vi "createElement.vi"(6 "collectionInfo":T1, 8 "error in (no error)":errorcluster, 9 "elementBasicType":string, 10 "elementName":string, 11 "ElementFactory in":refnum<class "ElementFactory.lvclass">) -> (0 "error out":errorcluster, 2 "element":refnum<class "Element.lvclass">, 3 "ElementFactory out":refnum<class "ElementFactory.lvclass">)   [LabVIEW 2016, in "ElementFactory.lvclass"]
uses:
  ElementFactory.lvclass
  Element/Element.lvclass
  Typedefs/CollectionInfo.ctl
  Elements/Primitive/Primitive.lvclass
  D:/Code/ts_SALLabVIEW/SALTypeGenerator/Element/Element.lvclass
  Elements/Short/Short.lvclass
  D:/Code/ts_SALLabVIEW/SALTypeGenerator/Elements/Primitive/Primitive.lvclass
  Elements/Long/Long.lvclass
  Elements/LongLong/LongLong.lvclass
  Elements/UnsignedShort/UnsignedShort.lvclass
  Elements/UnsignedLong/UnsignedLong.lvclass
  Elements/UnsignedLongLong/UnsignedLongLong.lvclass
  Elements/Float/Float.lvclass
  Elements/Double/Double.lvclass
  Elements/Char/Char.lvclass
  Elements/Boolean/Boolean.lvclass
  Elements/String/String.lvclass
  Elements/String/String.lvclass/String.ctl
  Elements/Array/Array.lvclass
  Elements/Array/Array.lvclass/Array.ctl
  Element/Element.lvclass/Element.ctl
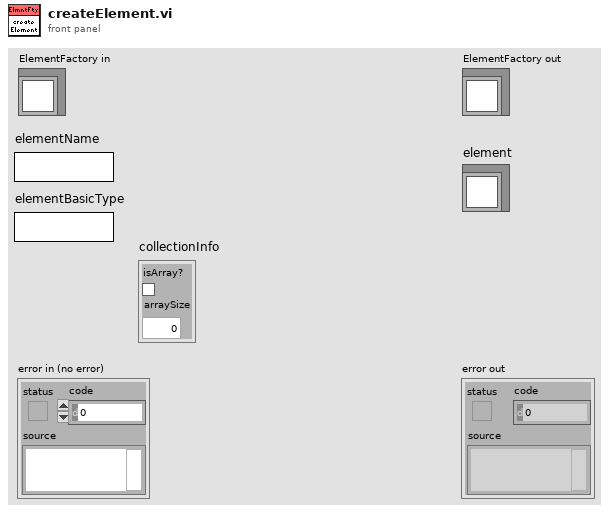
[diagram p1: front panel]
types:
  T1 = typedef "CollectionInfo.ctl" = cluster{"isArray?":bool, "arraySize":u16}
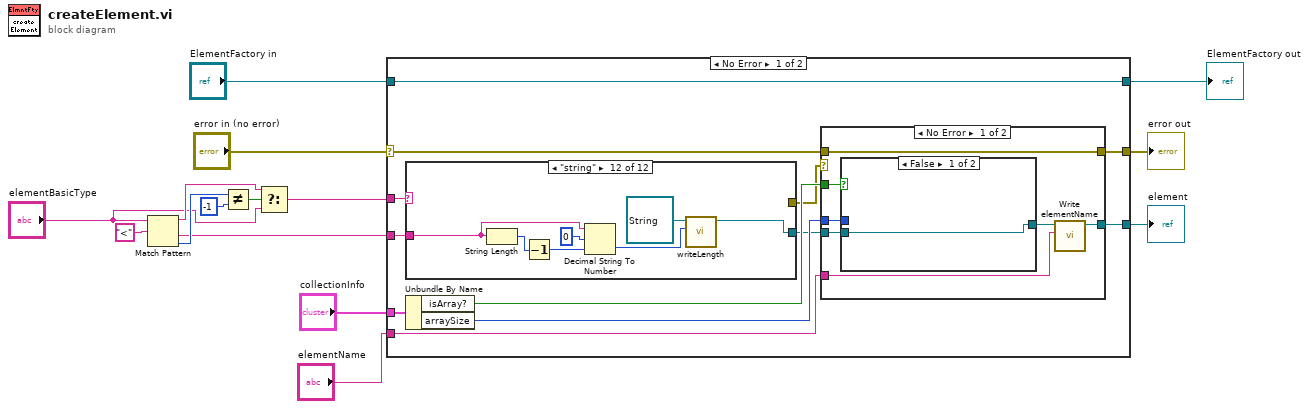
[diagram p0: block diagram]
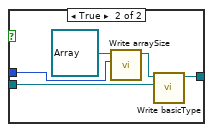
[diagram p2: hidden frame]
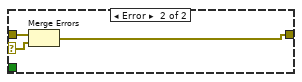
[diagram p3: hidden frame]
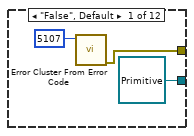
[diagram p4: hidden frame]
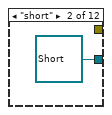
[diagram p5: hidden frame]
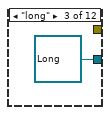
[diagram p6: hidden frame]
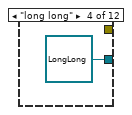
[diagram p7: hidden frame]
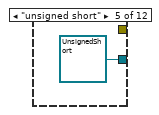
[diagram p8: hidden frame]
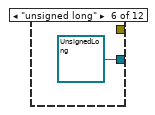
[diagram p9: hidden frame]
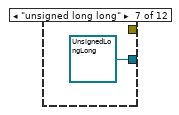
[diagram p10: hidden frame]
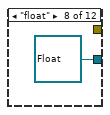
[diagram p11: hidden frame]
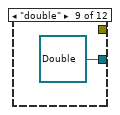
[diagram p12: hidden frame]
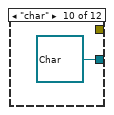
[diagram p13: hidden frame]
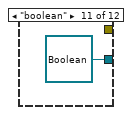
[diagram p14: hidden frame]
diagram:
  n1 = Match Pattern(string="elementBasicType", regular expression="<") -> (before substring=w4:string, after substring=w1:string, offset past match=w7:i32)  [unwired: 1 in, 1 out]
  n2 = Not Equal?(x=w7, y=-1) -> (x != y?=w5:bool)
  n3 = Select(t=w4, s=w5, f="elementBasicType") -> (s? t:f=w2:string)
  n4 = case shown="No Error" "error in (no error)" {
    selector: "error in (no error)" -> [w20 w65]
    tunnel: [w19 w65] -> w9
    tunnel: [w27 w64] -> w14
    tunnel: "ElementFactory in" -> [w27 w64]
    tunnel: w2 -> [w25 _]
    tunnel: "collectionInfo" -> [w26 _]
    tunnel: [w18 _] -> w13
    tunnel: "elementName" -> [w17 _]
    tunnel: w1 -> [w16 _]
    frame No Error {
      n5 = case shown="\"string\"" w25 {
        tunnel: [refnum<class "Primitive.lvclass"> refnum ("Boolean.lvclass") refnum<class "Short.lvclass"> refnum ("Short.lvclass") refnum<class "Long.lvclass"> refnum ("Long.lvclass") refnum<class "LongLong.lvclass"> refnum ("LongLong.lvclass") refnum<class "UnsignedShort.lvclass"> refnum ("UnsignedShort.lvclass") refnum<class "UnsignedLong.lvclass"> refnum ("UnsignedLong.lvclass") refnum<class "UnsignedLongLong.lvclass"> refnum ("UnsignedLongLong.lvclass") refnum<class "Float.lvclass"> refnum ("Float.lvclass") refnum<class "Double.lvclass"> refnum ("Double.lvclass") refnum<class "Char.lvclass"> refnum ("Char.lvclass") refnum<class "Boolean.lvclass"> refnum ("Boolean.lvclass") w58] -> w22
        tunnel: [w45 _ _ _ _ _ _ _ _ _ _ _] -> w21
        tunnel: w16 -> [_ _ _ _ _ _ _ _ _ _ _ w61]
        frame "False", Default {
          n6 = call <vilib>:"Error Cluster From Error Code.vi"("error code (0)"=5107) -> ("error out"=w45:errorcluster)  [unwired: 8 in]
        }
        frame "short" {
        }
        frame "long" {
        }
        frame "long long" {
        }
        frame "unsigned short" {
        }
        frame "unsigned long" {
        }
        frame "unsigned long long" {
        }
        frame "float" {
        }
        frame "double" {
        }
        frame "char" {
        }
        frame "boolean" {
        }
        frame "string" {
          n7 = String Length(string=w61) -> (length=w63:i32)
          n8 = Decrement(x=w63) -> (x-1=w62:i32)
          n9 = Decimal String To Number(string=w61, offset=0, default (0L)=w62) -> (number=w57:i32)  [unwired: 1 out]
          n10 = call "writeLength.vi"("Length"=w57, "String in"=refnum<class "String.lvclass"> refnum ("String.lvclass")) -> ("String out"=w58:refnum<class "String.lvclass">)  [unwired: 9 in]
        }
      }
      n11 = Unbundle By Name(w26) -> ("isArray?"=w23:bool, "arraySize"=w24:u16)
      n12 = case shown="No Error" w21 {
        selector: w21 -> [_ w42]
        tunnel: w24 -> [w34 _]
        tunnel: w23 -> [w33 _]
        tunnel: w22 -> [w32 _]
        tunnel: w20 -> [w31 w43]
        tunnel: [w31 w41] -> w19
        tunnel: [w29 _] -> w18
        tunnel: w17 -> [w28 _]
        frame No Error {
          n13 = case shown="False" w33 {
            tunnel: w34 -> [_ w39]
            tunnel: w32 -> [w35 w37]
            tunnel: [w35 w36] -> w30
            frame False {
            }
            frame True {
              n14 = call "Write arraySize.vi"("arraySize"=w39, "Array in"=refnum<class "Array.lvclass"> refnum ("Array.lvclass")) -> ("Array out"=w38:refnum<class "Array.lvclass">)  [unwired: 9 in]
              n15 = call "Write basicType.vi"("basicType"=w37, "Array in"=w38) -> ("Array out"=w36:refnum<class "Array.lvclass">)  [unwired: 9 in]
            }
          }
          n16 = call "Write elementName.vi"("elementName"=w28, "Element in"=w30) -> ("Element out"=w29:refnum<class "Element.lvclass">)  [unwired: 9 in]
        }
        frame Error {
          n17 = Merge Errors(w43, w42) -> (w41:errorcluster)
        }
      }
    }
    frame Error {
    }
  }
  "error out" <- w9
  "ElementFactory out" <- w14
  "element" <- w13
